vi "例4-5.vi"() -> ()   [LabVIEW 2019]
panel:
  out "Sqrt":dbl format="%_5g"
  in  "X":dbl=2.0
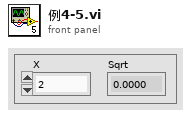
[diagram p1: front panel]
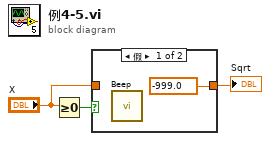
[diagram p0: block diagram]
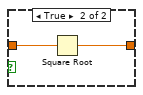
[diagram p2: hidden frame]
diagram:
  n1 = Greater Or Equal To 0?(x="X") -> (x >= 0?=w3:bool)
  n2 = case shown="假" w3 {
    tunnel: "X" -> [_ w6]
    tunnel: [-999.0 w5] -> w1
    frame False {
      n3 = call <vilib>:"Beep.vi"() -> ()  [unwired: 12 in]
    }
    frame True {
      n4 = Square Root(x=w6) -> (sqrt(x)=w5:dbl)
    }
  }
  "Sqrt" <- w1
